vi "ex6-8.vi"   [LabVIEW 2013]
uses:
  <vilib>/NXT/Subs/MotorOutput.ctl
  <vilib>/NXT/Block Support/NXT_InputPort.ctl
  <vilib>/NXT/Block Support/NXT_ButtonSelector.ctl
  <vilib>/NXT/Dual Mode Library/Sensors/Light_On.vi
  <vilib>/NXT/Dual Mode Library/Motors/MotorBrake.vi
  <vilib>/NXT/Dual Mode Library/Sensors/readNXTButton.vi
  <vilib>/NXT/Dual Mode Library/Waits/Wait_Num(msec).vi
  <vilib>/NXT/Dual Mode Library/Motors/MotorOn.vi
types:
  T1 = typedef "MotorOutput.ctl" = u8
  T2 = typedef "NXT_InputPort.ctl" = u32
  T3 = typedef "NXT_ButtonSelector.ctl" = u16
  T4 = typedef "LVHSConnector.ctl" = refnum<class "BrickReference.lvclass">
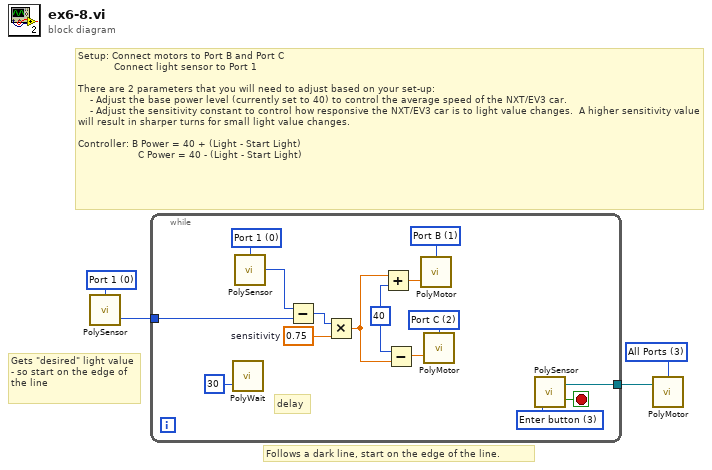
[diagram p0: block diagram]
diagram:
  w4 = T1 3 items=["Port A"=0, "Port B"=1, "Port C"=2, "Ports A & B"=4, "Ports A & C"=5, "Ports B & C"=6, "All Ports"=3] ("Port (All Ports)")
  w1 = T2 0 items=["Port 1", "Port 2", "Port 3", "Port 4"] ("Input Port (Port 3)")
  # "Gets \"desired\" light value - so start on the edge of the line"
  # "Follows a dark line, start on the edge of the line."
  # "Setup: Connect motors to Port B and Port C\n            Connect light sensor to Port 1\n\nThere are 2 parameters that you will need to adjust based on your set-up:  \n    - Adjust the base power level (currently set to 40) to control the average speed of the NXT/EV3 car.\n    - Adjust the sensitivity constant to control how responsive the NXT/EV3 car is to light value changes.  A higher sensitivity value will result in sharper turns for small light value changes. \n \nController: B Power = 40 + (Light - Start Light)\n                    C Power = 40 - (Light - Start Light)"
  n1 = call-poly <vilib>:"PolySensor.vi"("Port (Port 3)"=w1) -> ("Scaled Value"=w2:i16)  [unwired: 1 in, 2 out]
  n2 = while {
    tunnel: w2 -> [w14]
    tunnel: [w7] -> w3
    stop <- w13 stop-if-true
    w5 = T1 2 items=["Port A"=0, "Port B"=1, "Port C"=2, "Ports A & B"=4, "Ports A & C"=5, "Ports B & C"=6, "All Ports"=3] ("Output Port (All Ports)")
    w6 = T1 1 items=["Port A"=0, "Port B"=1, "Port C"=2, "Ports A & B"=4, "Ports A & C"=5, "Ports B & C"=6, "All Ports"=3] ("Output Port (All Ports)")
    w8 = sgl 0.75  # sensitivity
    w12 = T3 3 items=["Enter button"=3, "Left button"=2, "Right button"=1] ("Button (Enter button)")
    w16 = 40 ("y")
    w19 = T2 0 items=["Port 1", "Port 2", "Port 3", "Port 4"] ("Input Port (Port 3)")
    # "delay"
    n3 = call-poly <vilib>:"PolyWait.vi"("Time (100 msec)"=u32 30 ("Time (1 sec)")) -> ()  [unwired: 3 in, 1 out]
    n4 = call-poly <vilib>:"PolySensor.vi"("Port (Port 3)"=w19) -> ("Scaled Value"=w18:i16)  [unwired: 1 in, 2 out]
    n5 = Subtract(x=w18, y=w14) -> (x-y=w10:i16)
    n6 = Multiply(x=w10, y=w8) -> (x*y=w9:sgl)
    n7 = Add(x=w9, y=w16) -> (x+y=w17:sgl)
    n8 = Subtract(x=w16, y=w9) -> (x-y=w15:sgl)
    n9 = call-poly <vilib>:"PolyMotor.vi"("Power (75)"=w17, "Output Port (All Ports)"=w6) -> ()  [unwired: 1 in, 2 out]
    n10 = call-poly <vilib>:"PolyMotor.vi"("Power (75)"=w15, "Output Port (All Ports)"=w5) -> ()  [unwired: 1 in, 2 out]
    n11 = call-poly <vilib>:"PolySensor.vi"("Button (Enter button)"=w12) -> ("Yes/No"=w13:bool, "NXT/EV3"=w7:T4)  [unwired: 1 in, 1 out]
  }
  n12 = call-poly <vilib>:"PolyMotor.vi"("NXT/EV3"=w3, "Port (All Ports)"=w4) -> ()  [unwired: 3 out]
